vi "ParseBS.vi"(11 "BS String":string) -> (1 "Y Pos":dbl, 2 "X Pos":dbl, 3 "Target Locations":dbl[][](array[numeric]))   [LabVIEW 2012]
panel:
  out "number 2":dbl
  out "number":dbl
  out "String":string
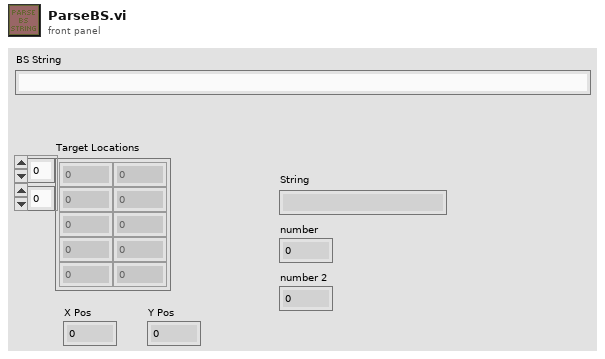
[diagram p1: front panel]
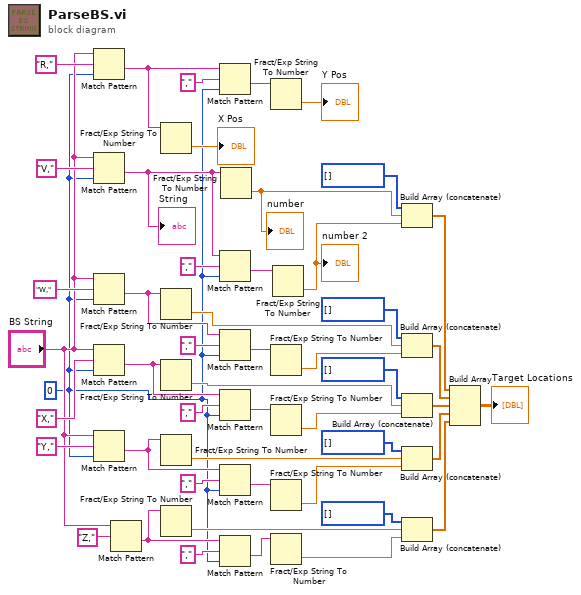
[diagram p0: block diagram]
diagram:
  w1 = 0 ("offset (0)")
  n1 = Match Pattern(string="BS String", regular expression="R,", offset (0)=w1) -> (after substring=w13:string)  [unwired: 3 out]
  n2 = Match Pattern(string="BS String", regular expression="V,", offset (0)=w1) -> (after substring=w39:string)  [unwired: 3 out]
  "String" <- w39
  n3 = Match Pattern(string="BS String", regular expression="W,", offset (0)=w1) -> (after substring=w38:string)  [unwired: 3 out]
  n4 = Match Pattern(string="BS String", regular expression="X,", offset (0)=w1) -> (after substring=w28:string)  [unwired: 3 out]
  n5 = Match Pattern(string="BS String", regular expression="Y,", offset (0)=w1) -> (after substring=w25:string)  [unwired: 3 out]
  n6 = Match Pattern(string="BS String", regular expression="Z,") -> (after substring=w7:string)  [unwired: 1 in, 3 out]
  n7 = Fract/Exp String To Number(string=w13) -> (number=→"X Pos":dbl)  [unwired: 3 in, 1 out]
  n8 = Fract/Exp String To Number(string=w38) -> (number=w31:dbl)  [unwired: 3 in, 1 out]
  n9 = Fract/Exp String To Number(string=w28) -> (number=w22:dbl)  [unwired: 3 in, 1 out]
  n10 = Fract/Exp String To Number(string=w25) -> (number=w20:dbl)  [unwired: 3 in, 1 out]
  n11 = Fract/Exp String To Number(string=w7) -> (number=w6:dbl)  [unwired: 3 in, 1 out]
  n12 = Match Pattern(string=w13, regular expression=",", offset (0)=w1) -> (after substring=w14:string)  [unwired: 3 out]
  n13 = Match Pattern(string=w39, regular expression=",", offset (0)=w1) -> (after substring=w40:string)  [unwired: 3 out]
  n14 = Match Pattern(string=w38, regular expression=",", offset (0)=w1) -> (after substring=w43:string)  [unwired: 3 out]
  n15 = Match Pattern(string=w28, regular expression=",", offset (0)=w1) -> (after substring=w44:string)  [unwired: 3 out]
  n16 = Match Pattern(string=w25, regular expression=",", offset (0)=w1) -> (after substring=w26:string)  [unwired: 3 out]
  n17 = Match Pattern(string=w7, regular expression=",", offset (0)=w1) -> (after substring=w8:string)  [unwired: 3 out]
  n18 = Fract/Exp String To Number(string=w39) -> (number=w36:dbl)  [unwired: 3 in, 1 out]
  "number" <- w36
  n19 = Fract/Exp String To Number(string=w14) -> (number=→"Y Pos":dbl)  [unwired: 3 in, 1 out]
  n20 = Fract/Exp String To Number(string=w43) -> (number=w30:dbl)  [unwired: 3 in, 1 out]
  n21 = Fract/Exp String To Number(string=w44) -> (number=w21:dbl)  [unwired: 3 in, 1 out]
  n22 = Fract/Exp String To Number(string=w26) -> (number=w19:dbl)  [unwired: 3 in, 1 out]
  n23 = Fract/Exp String To Number(string=w8) -> (number=w5:dbl)  [unwired: 3 in, 1 out]
  n24 = Fract/Exp String To Number(string=w40) -> (number=w35:dbl)  [unwired: 3 in, 1 out]
  "number 2" <- w35
  n25 = Build Array (concatenate)(i32[] [], w36, w35) -> (w34:dbl[])
  n26 = Build Array (concatenate)(i32[] [], w31, w30) -> (w29:dbl[])
  n27 = Build Array (concatenate)(i32[] [], w22, w21) -> (w18:dbl[])
  n28 = Build Array (concatenate)(i32[] [], w20, w19) -> (w17:dbl[])
  n29 = Build Array (concatenate)(i32[] [], w6, w5) -> (w3:dbl[])
  n30 = Build Array(w34, w29, w18, w17, w3) -> (→"Target Locations":dbl[][])
